vi "view_wf.vi"() -> ()   [LabVIEW 2013]
uses:
  <vilib>/Utility/xml.llb/Read From XML File(string).vi
panel:
  out "correction":waveform(dbl)(graph)
  out "electrodes":waveform(dbl)[](graph)=[{"t0"=timestamp(0 s since 1904-01-01), "dt"=5e-08, "Y"=array[2000 elements]}, {"t0"=timestamp(0 s since 1904-01-01), "dt"=5e-08, "Y"=array[2000 elements]}, {"t0"=timestamp(0 s since 1904-01-01), "dt"=5e-08, "Y"=array[2000 elements]}, {"t0"=timestamp(0 s since 1904-01-01), "dt"=5e-08, "Y"=array[2000 elements]}, {"t0"=timestamp(0 s since 1904-01-01), "dt"=5e-08, "Y"=array[2000 elements]}]
  # "Plot a *.wf (XML) file.  Run for file prompt."
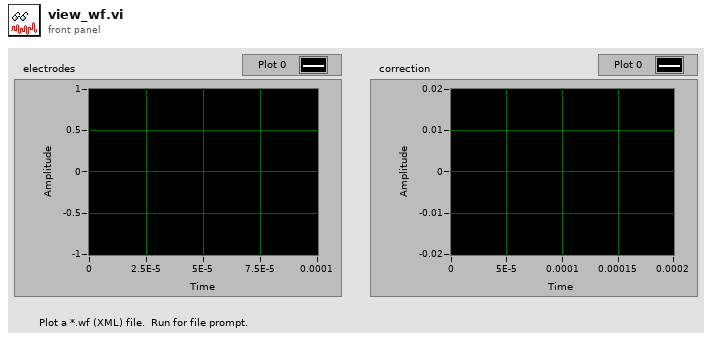
[diagram p1: front panel]
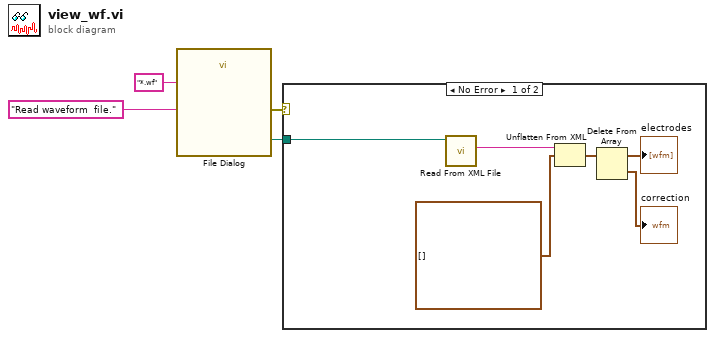
[diagram p0: block diagram]
diagram:
  n1 = call "File Dialog"("prompt"="Read waveform  file.", "pattern (all files)"="*.wf" ("pattern label")) -> ("selected path"=w2:path, "error out"=w1:errorcluster)  [unwired: 10 in, 2 out]
  n2 = case shown="No Error" w1 {
    tunnel: w2 -> [w10 _]
    frame No Error {
      n3 = call-poly <vilib>:"Read From XML File.vi"("XML File Path"=w10) -> ("XML Elements"=w9:string)  [unwired: 8 in, 2 out]
      n4 = Unflatten From XML(xml string=w9, type=waveform(dbl)[] [] ("electrodes 2")) -> (value=w7:waveform(dbl)[])  [unwired: 1 in, 1 out]
      n5 = Delete From Array(array=w7) -> (deleted portion=→"correction":waveform(dbl), array with subset deleted=→"electrodes":waveform(dbl)[])  [unwired: 2 in]
    }
    frame Error {
    }
  }
